vi "YawHistoryGlobal.vi"(9 "Initialize":bool, 10 "Yaw":dbl, 11 "Update":bool) -> (3 "Average Yaw History":dbl)   [LabVIEW 2014, in "Nav6.lvlib"]
uses:
  Nav6.lvlib
panel:
  out "Index":u8
  out "Yaw History":dbl[](array[numeric])
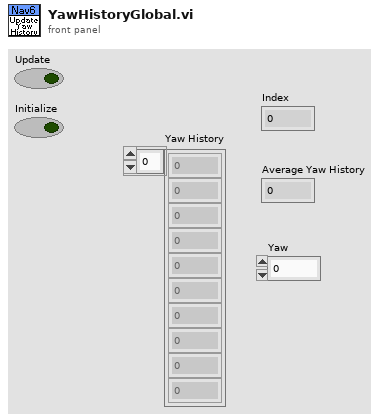
[diagram p1: front panel]
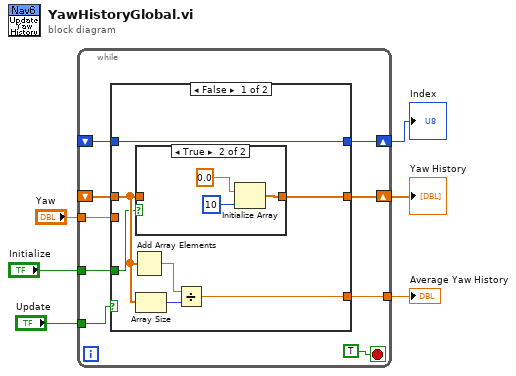
[diagram p0: block diagram]
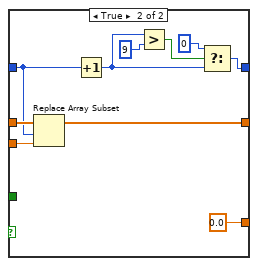
[diagram p3: hidden frame]
diagram:
  n1 = while {
    tunnel: "Update" -> [w14]
    tunnel: "Yaw" -> [w13]
    shift-right: [w10] -> w3
    shift-left: _ -> [w11]
    tunnel: [w9] -> w4
    shift-right: [w8] -> w2
    shift-left: _ -> [w12]
    tunnel: "Initialize" -> [w7]
    stop <- TRUE stop-if-true
    n2 = case shown="False" w14 {
      tunnel: w13 -> [_ w36]
      tunnel: w12 -> [w19 w32]
      tunnel: w11 -> [w18 w35]
      tunnel: [w17 w34] -> w10
      tunnel: [w20 0.0] -> w9
      tunnel: [w19 w27] -> w8
      tunnel: w7 -> [w16 _]
      frame False {
        n3 = Add Array Elements(numeric array=w18) -> (sum=w22:dbl)
        n4 = case shown="True" w16 {
          tunnel: w18 -> [w23 _]
          tunnel: [w23 w26] -> w17
          frame False {
          }
          frame True {
            n5 = Initialize Array(0.0 ("element"), 10 ("dimension size")) -> (w26:dbl[])
          }
        }
        n6 = Array Size(array=w18) -> (size(s)=w21:i32)
        n7 = Divide(x=w22, y=w21) -> (x/y=w20:dbl)
      }
      frame True {
        n8 = Replace Array Subset(array=w35, new element=w36, index=w32) -> (w34:dbl[])
        n9 = Increment(x=w32) -> (x+1=w28:u8)
        n10 = Greater?(x=w28, y=u8 9) -> (0:w30:bool)
        n11 = Select(t=u8 0, s=w30, f=w28) -> (s? t:f=w27:u8)
      }
    }
  }
  "Yaw History" <- w3
  "Index" <- w2
  "Average Yaw History" <- w4
